vi "tm_getframe_a.vi"(8 "error in (no error)":errorcluster, 9 "Frame Index":i32=-1, 10 "Buffer":T1, 11 "Handle in":u32) -> (0 "error out":errorcluster, 1 "Data 8":u8[][](array[numeric]), 2 "Data 16":u16[][](array[numeric]), 3 "Handle out":u32)   [LabVIEW 2015]
uses:
  tmcamcon.dll
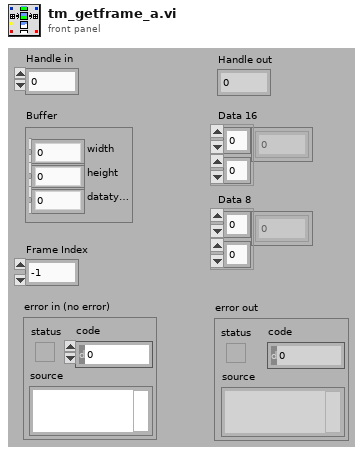
[diagram p1: front panel]
types:
  T1 = cluster{"width":u32, "height":u32, "datatype":u32}
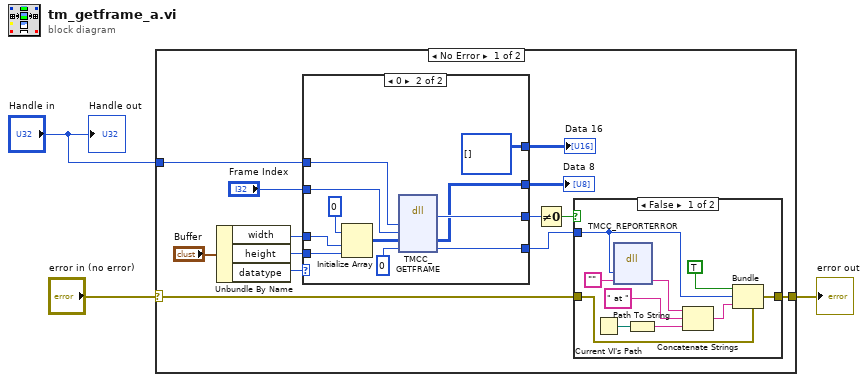
[diagram p0: block diagram]
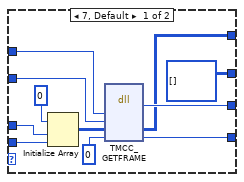
[diagram p2: hidden frame]
diagram:
  n1 = case shown="No Error" "error in (no error)" {
    selector: "error in (no error)" -> [w15 w50]
    tunnel: [w14 w50] -> w2
    tunnel: "Handle in" -> [w13 _]
    frame No Error {
      n2 = Unbundle By Name("Buffer") -> ("width"=w6:u32, "height"=w5:u32, "datatype"=w4:u32)
      n3 = case shown="0" w4 {
        tunnel: w6 -> [w26 w37]
        tunnel: w5 -> [w25 w36]
        tunnel: w13 -> [w24 w35]
        tunnel: "Frame Index" -> [w21 w32]
        tunnel: [w20 w31] -> w11
        tunnel: [w19 w30] -> w10
        tunnel: [u8[][] [] ("Data 8") w28] -> w9
        tunnel: [w17 u16[][] [] ("Data 16")] -> w8
        frame 7, Default {
          n4 = Initialize Array(u16 0, w26, w25) -> (w22:u16[][])
          n5 = dll-call lib="tmcamcon.dll" fn="TMCC_GETFRAME"("index"=w24, "frameindex"=w21, "imgarray"=w22, "Erval"=0) -> ("return type"=w19:u32, "imgarray"=w17:u16[][], "Erval"=w20:i32)  [unwired: 5 in, 2 out]
        }
        frame 0 {
          n6 = Initialize Array(u8 0, w37, w36) -> (w33:u8[][])
          n7 = dll-call lib="tmcamcon.dll" fn="TMCC_GETFRAME"("index"=w35, "frameindex"=w32, "imgarray"=w33, "Erval"=0) -> ("return type"=w30:u32, "imgarray"=w28:u8[][], "Erval"=w31:i32)  [unwired: 5 in, 2 out]
        }
      }
      "Data 16" <- w8
      "Data 8" <- w9
      n8 = Not Equal To 0?(x=w10) -> (x != 0?=w16:bool)
      n9 = case shown="False" w16 {
        tunnel: w15 -> [w48 w49]
        tunnel: [w47 w49] -> w14
        tunnel: w11 -> [w41 _]
        frame False {
          n10 = Current VI's Path() -> (path=w46:path)
          n11 = dll-call lib="tmcamcon.dll" fn="TMCC_REPORTERROR"("error"=w41, "buf"="") -> ("buf"=w40:string)  [unwired: 5 in, 2 out]
          n12 = Path To String(path=w46) -> (string=w42:string)
          n13 = Concatenate Strings(w40, " at ", w42) -> (w45:string)
          n14 = Bundle(cluster=w48, "status"=TRUE, "code"=w41, "source"=w45) -> (w47:errorcluster)
        }
        frame True {
        }
      }
    }
    frame Error {
    }
  }
  "error out" <- w2
  "Handle out" <- "Handle in"
